vi "例4-19（全局变量）.vi"() -> ()   [LabVIEW 2019]
panel:
  in  "数值传递":dbl
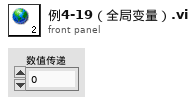
[diagram p1: front panel]
diagram:
